vi "Tegam4040_Offset_Cal.vi"(9 "Waveform Array":waveform(dbl)[](array[waveform]), 11 "Digitizer Range":dbl) -> (0 "Tegam#2 True Offset":dbl, 1 "Tegam#2 Predicted DAC":dbl, 2 "Tegam#1 True Offset":dbl, 3 "Tegam#1 Predicted DAC":dbl)   [LabVIEW 2010]
uses:
  Tegam4040_Offset_Global.vi
  <vilib>/Analysis/NI_AALBase.lvlib
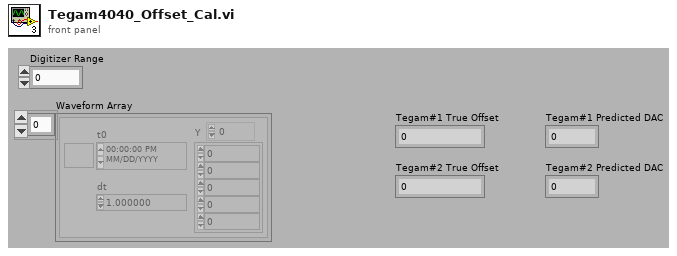
[diagram p1: front panel]
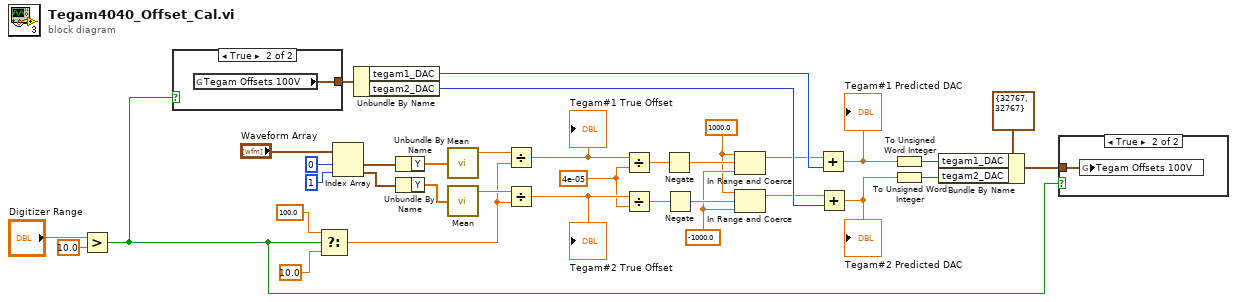
[diagram p0: block diagram]
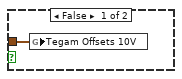
[diagram p2: hidden frame]
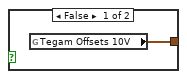
[diagram p3: hidden frame]
diagram:
  w11 = -1000.0 ("tegam1_DAC")
  w10 = 1000.0 ("tegam1_DAC")
  w1 = 4e-05 ("f")
  n1 = Greater?(x="Digitizer Range", y=10.0) -> (0:w4:bool)
  n2 = case shown="True" w4 {
    tunnel: [w36 w37] -> w5
    frame False {
      n3 = global read "Tegam4040_Offset_Global.vi" "Tegam Offsets 10V"() -> (w36:cluster{"tegam2_DAC":u16, "tegam1_DAC":u16})
    }
    frame True {
      n4 = global read "Tegam4040_Offset_Global.vi" "Tegam Offsets 100V"() -> (w37:cluster{"tegam2_DAC":u16, "tegam1_DAC":u16})
    }
  }
  n5 = Select(t=100.0, s=w4, f=10.0) -> (s? t:f=w2:dbl)
  n6 = Index Array(array="Waveform Array", index #1=0 ("index"), index #2=1 ("index")) -> (element #1=w32:waveform(dbl), element #2=w33:waveform(dbl))
  n7 = Unbundle By Name(w5) -> ("tegam1_DAC"=w15:u16, "tegam2_DAC"=w14:u16)
  n8 = Unbundle By Name(w32) -> ("Y"=w31:dbl[])
  n9 = Unbundle By Name(w33) -> ("Y"=w29:dbl[])
  n10 = call <vilib>:"Mean.vi"("X"=w31) -> ("mean"=w26:dbl)  [unwired: 1 out]
  n11 = call <vilib>:"Mean.vi"("X"=w29) -> ("mean"=w25:dbl)  [unwired: 1 out]
  n12 = Divide(x=w26, y=w2) -> (x/y=w24:dbl)
  "Tegam#1 True Offset" <- w24
  n13 = Divide(x=w25, y=w2) -> (x/y=w23:dbl)
  "Tegam#2 True Offset" <- w23
  n14 = Divide(x=w24, y=w1) -> (x/y=w21:dbl)
  n15 = Divide(x=w23, y=w1) -> (x/y=w22:dbl)
  n16 = Negate(x=w21) -> (-x=w12:dbl)
  n17 = Negate(x=w22) -> (-x=w13:dbl)
  n18 = In Range and Coerce(upper limit=w10, x=w12, lower limit=w11) -> (coerced(x)=w9:dbl)  [unwired: 1 out]
  n19 = In Range and Coerce(upper limit=w10, x=w13, lower limit=w11) -> (coerced(x)=w8:dbl)  [unwired: 1 out]
  n20 = Add(x=w9, y=w15) -> (x+y=w19:dbl)
  "Tegam#1 Predicted DAC" <- w19
  n21 = Add(x=w8, y=w14) -> (x+y=w16:dbl)
  "Tegam#2 Predicted DAC" <- w16
  n22 = To Unsigned Word Integer(number=w19) -> (unsigned 16bit integer=w17:u16)
  n23 = To Unsigned Word Integer(number=w16) -> (unsigned 16bit integer=w18:u16)
  n24 = Bundle By Name(cluster=cluster{"tegam2_DAC":u16, "tegam1_DAC":u16} {"tegam2_DAC"=32767, "tegam1_DAC"=32767} ("Tegam Offsets"), "tegam1_DAC"=w17, "tegam2_DAC"=w18) -> (w3:cluster{"tegam2_DAC":u16, "tegam1_DAC":u16})
  n25 = case shown="True" w4 {
    tunnel: w3 -> [w38 w39]
    frame False {
      n26 = global write "Tegam4040_Offset_Global.vi" "Tegam Offsets 10V"(w38) -> ()
    }
    frame True {
      n27 = global write "Tegam4040_Offset_Global.vi" "Tegam Offsets 100V"(w39) -> ()
    }
  }
